vi "UpdateHeaterDC.vi"(7 "LVWSR":refnum<class "Web Request.lvclass">, 10 "dc":u8, 11 "heater_id":string) -> ()   [LabVIEW 2017]
uses:
  <vilib>/wsapi/Web Request.lvclass
  Controller/Messages/Update Heater DC MSG/Update Heater DC MSG.lvclass
  C:/Program Files (x86)/National Instruments/LabVIEW 2017/vi.lib/ActorFramework/Message/Message.lvclass
  <vilib>/ActorFramework/Message Enqueuer/Message Enqueuer.lvclass/Message Enqueuer.ctl
  <vilib>/ActorFramework/Message Priority Queue/Priority Enqueue.vi
  Controller/gController.lvclass
  <vilib>/ActorFramework/Message Enqueuer/Message Enqueuer.lvclass
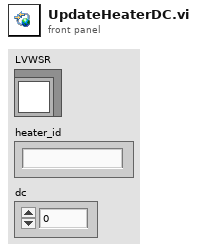
[diagram p1: front panel]
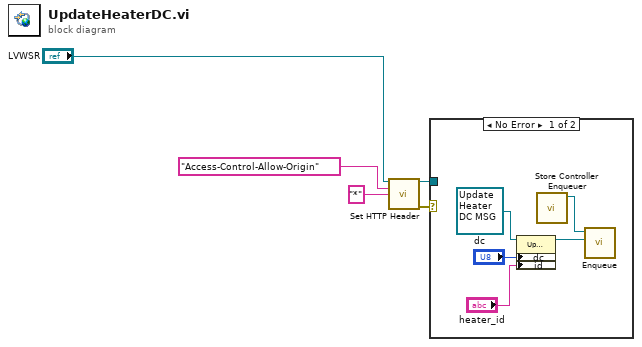
[diagram p0: block diagram]
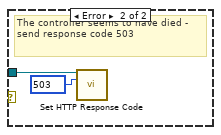
[diagram p2: hidden frame]
diagram:
  n1 = call <vilib>:"Set HTTP Header.vi"("LabVIEW Web Service Request"="LVWSR", "header"="Access-Control-Allow-Origin", "header value"="*") -> ("LabVIEW Web Service Request out"=w3:refnum<class "Web Request.lvclass">, "error out"=w2:errorcluster)  [unwired: 11 in]
  n2 = case shown="No Error" w2 {
    tunnel: w3 -> [_ w11]
    frame No Error {
      n3 = property class="Update Heater DC MSG.lvclass"(reference=refnum<class "Update Heater DC MSG.lvclass"> refnum ("Controller.lvlib:Update Heater DC MSG.lvclass"), "dc"="dc", "id"="heater_id") -> (reference out=w9:refnum<class "Update Heater DC MSG.lvclass">)  [unwired: 1 in, 1 out]
      n4 = call "Store Controller Enqueuer.vi"() -> ("Controller Enqueuer Out"=w10:refnum<class "Message Enqueuer.lvclass">)  [unwired: 11 in]
      n5 = call <vilib>:"Enqueue.vi"("Message"=w9, "Message Enqueuer in"=w10) -> ()  [unwired: 8 in, 2 out]
    }
    frame Error {
      w12 = 503 items=["100"=100, "101"=101, "200"=200, "201"=201, "202"=202, "203"=203, "204"=204, "205"=205, "206"=206, "300"=300, "301"=301, "302"=302, "303"=303, "304"=304, "305"=305, "306"=306, "307"=307, "400"=400, "401"=401, "402"=402, "403"=403, "404"=404, "405"=405, "406"=406, "407"=407, "408"=408, "409"=409, "410"=410, "411"=411, "412"=412, "413"=413, "414"=414, "415"=415, "416"=416, "417"=417, "500"=500, "501"=501, "502"=502, "503"=503, "504"=504, "505"=505] ("response code (200)")
      # "The controller seems to have died - send response code 503"
      n6 = call <vilib>:"Set HTTP Response Code.vi"("LabVIEW Web Service Request"=w11, "response code (200)"=w12) -> ()  [unwired: 12 in, 2 out]
    }
  }
